vi "Function.vi"(8 "error in (no error)":errorcluster, 10 "Boolean A":bool, 11 "One Terminal in":refnum<class "AbsFunc_One Term_Bool.lvclass">) -> (0 "error out":errorcluster, 2 "Boolean":bool, 3 "One Terminal out":refnum<class "AbsFunc_One Term_Bool.lvclass">)   [LabVIEW 2021, in "AbsFunc_One Term_Bool.lvclass"]
uses:
  AbsFunc_One Term_Bool.lvclass
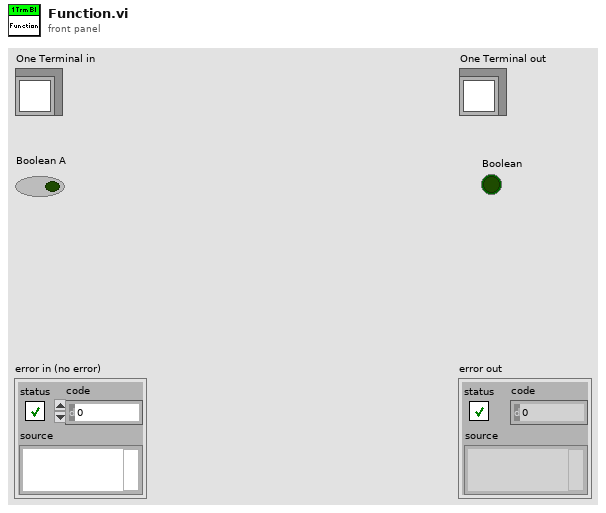
[diagram p1: front panel]
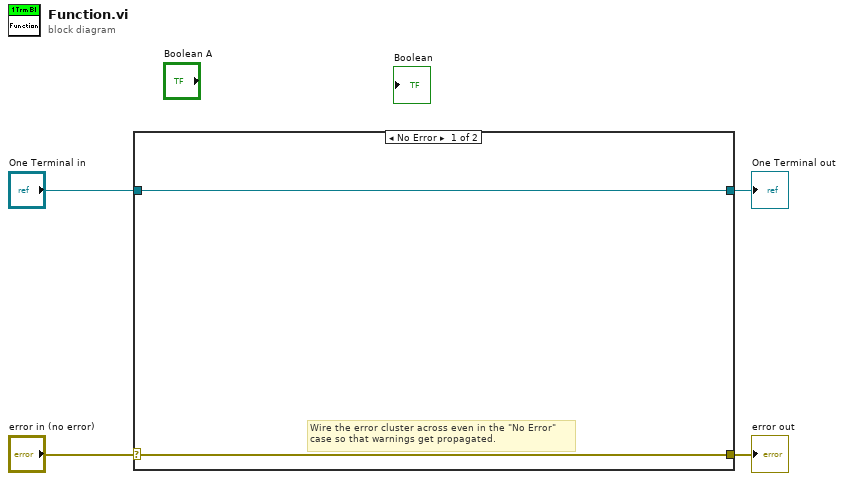
[diagram p0: block diagram]
diagram:
  n1 = case shown="No Error" "error in (no error)" {
    selector: "error in (no error)" -> [w5 w8]
    tunnel: [w5 w8] -> w3
    tunnel: [w6 w7] -> w1
    tunnel: "One Terminal in" -> [w6 w7]
    frame No Error {
      # "Wire the error cluster across even in the \"No Error\"\ncase so that warnings get propagated."
    }
    frame Error {
    }
  }
  "error out" <- w3
  "One Terminal out" <- w1
